vi "ADC_Start.vi"(8 "error in (no error)":errorcluster) -> (0 "error out":errorcluster, 3 "function return":i16)   [LabVIEW 2013, in "MeasurmentRoutines.lvlib"]
doc: "Description: This routine writes any new instrument setting information to the hardware and then starts the measurement. If the hardware is already measuring, this measurement is aborted. Previous measured data is lost\nInput: -\nOutput: Return value E_NOT_INITIALIZED | E_NO_ERRORS | E_NO_HARDWARE\n\nFunction prototype: word ADC_Start( void )\n\n\n\n\n\n\n\n\nshort int ADC_Start ( void );"
uses:
  MeasurmentRoutines.lvlib
  hs3.dll
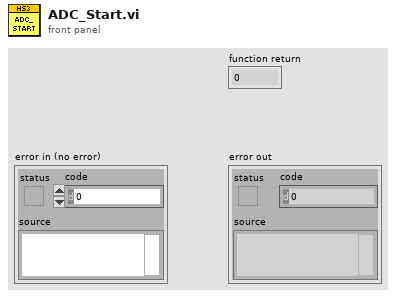
[diagram p1: front panel]
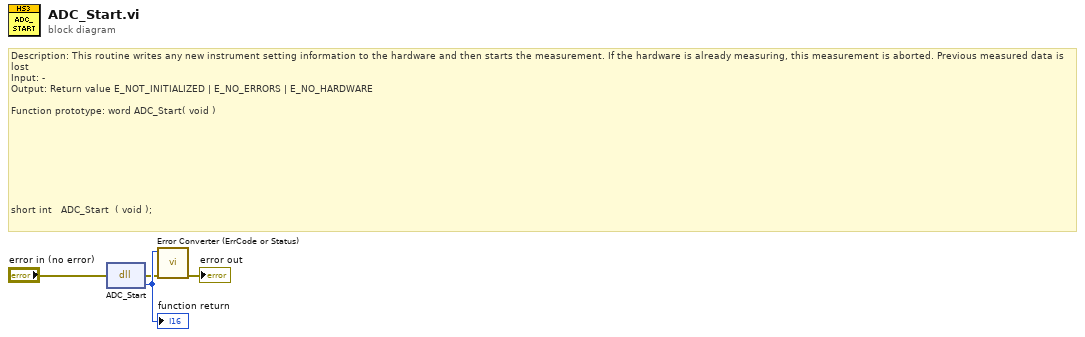
[diagram p0: block diagram]
diagram:
  # "Description: This routine writes any new instrument setting information to the hardware and then starts the measurement. If the hardware is already measuring, this measurement is aborted. Previous measured data is lost\nInput: -\nOutput: Return value E_NOT_INITIALIZED | E_NO_ERRORS | E_NO_HARDWARE\n\nFunction prototype: word ADC_Start( void )\n\n\n\n\n\n\n\n\nshort int \t\tADC_Start\t\t( void );"
  n1 = dll-call lib="C:/Documents and Settings/admin/Pulpit/HS3 LabViewLib/HS3_WRAPPER/hs3.*" fn="ADC_Start"(error in="error in (no error)") -> (error out=w2:errorcluster, w4:i16)  [unwired: 2 in, 1 out]
  "function return" <- w4
  n2 = call "Error Converter (ErrCode or Status).vi"("error in (no error)"=w2, "error code"=w4) -> ("error out"=→"error out":errorcluster)  [unwired: 9 in]
